vi "RichTextBoxExample.vi"   [LabVIEW 2017]
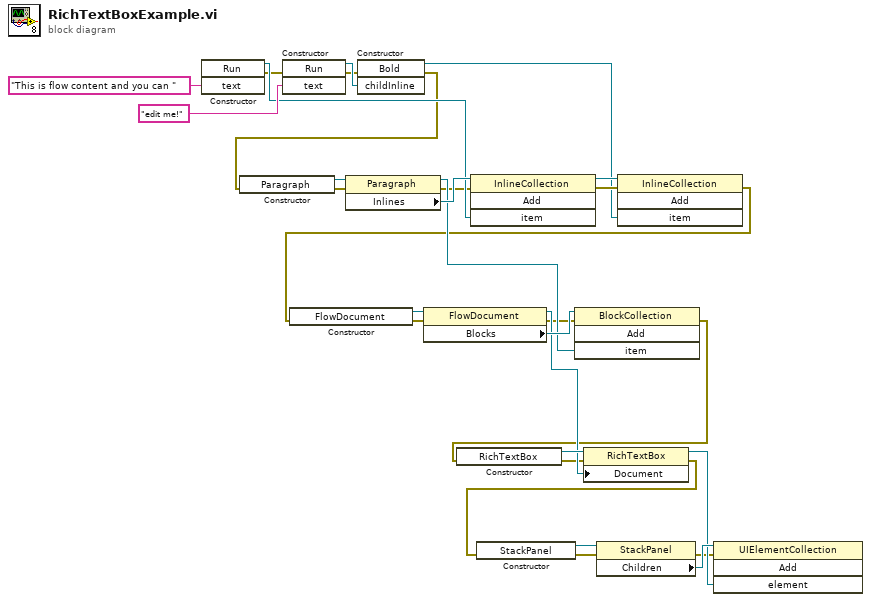
[diagram p0: block diagram]
diagram:
  n1 = constructor class="Run"("text"="This is flow content and you can ") -> (reference out=w24:refnum<k24>, error out=w4:errorcluster)  [unwired: 3 in, 2 out]
  n2 = constructor class="Run"(error in=w4, "text"="edit me!") -> (reference out=w30:refnum<k24>, error out=w3:errorcluster)  [unwired: 2 in, 2 out]
  n3 = constructor class="Bold"(error in=w3, "childInline"=w30) -> (reference out=w21:refnum<k24>, error out=w2:errorcluster)  [unwired: 2 in, 2 out]
  n4 = constructor class="Paragraph"(error in=w2) -> (reference out=w27:refnum<k24>, error out=w26:errorcluster)  [unwired: 2 in, 1 out]
  n5 = property class="Paragraph"(reference=w27, error in=w26) -> (reference out=w18:refnum<k24>, error out=w1:errorcluster, "Inlines"=w25:refnum<k24>)
  n6 = invoke class="InlineCollection" method="Add"(reference=w25, error in=w1, "item"=w24) -> (reference out=w23:refnum<k24>, error out=w22:errorcluster)  [unwired: 1 in, 2 out]
  n7 = invoke class="InlineCollection" method="Add"(reference=w23, error in=w22, "item"=w21) -> (error out=w7:errorcluster)  [unwired: 1 in, 3 out]
  n8 = constructor class="FlowDocument"(error in=w7) -> (reference out=w20:refnum<k24>, error out=w6:errorcluster)  [unwired: 2 in, 1 out]
  n9 = property class="FlowDocument"(reference=w20, error in=w6) -> (reference out=w16:refnum<k24>, error out=w5:errorcluster, "Blocks"=w19:refnum<k24>)
  n10 = invoke class="BlockCollection" method="Add"(reference=w19, error in=w5, "item"=w18) -> (error out=w11:errorcluster)  [unwired: 1 in, 3 out]
  n11 = constructor class="RichTextBox"(error in=w11) -> (reference out=w17:refnum<k24>, error out=w10:errorcluster)  [unwired: 2 in, 1 out]
  n12 = property class="RichTextBox"(reference=w17, error in=w10, "Document"=w16) -> (reference out=w13:refnum<k24>, error out=w9:errorcluster)
  n13 = constructor class="StackPanel"(error in=w9) -> (reference out=w15:refnum<k24>, error out=w12:errorcluster)  [unwired: 2 in, 1 out]
  n14 = property class="StackPanel"(reference=w15, error in=w12) -> (error out=w8:errorcluster, "Children"=w14:refnum<k24>)  [unwired: 1 out]
  n15 = invoke class="UIElementCollection" method="Add"(reference=w14, error in=w8, "element"=w13) -> ()  [unwired: 1 in, 4 out]
